vi "Set_Output.vi"(8 "error in (no error)":errorcluster caption="entrée d'erreur (pas d'erreur)", 10 "Output":string, 11 "Process (Default) en entrée":refnum<class "Process (Default).lvclass">) -> (0 "error out":errorcluster caption="sortie d'erreur", 3 "Process (Default) en sortie":refnum<class "Process (Default).lvclass">)   [LabVIEW 2020, in "Library Instrument & Equipement.lvlib" / "Process (Default).lvclass"]
uses:
  Process (Default).lvclass
  Process (Default).lvclass/Process (Default).ctl
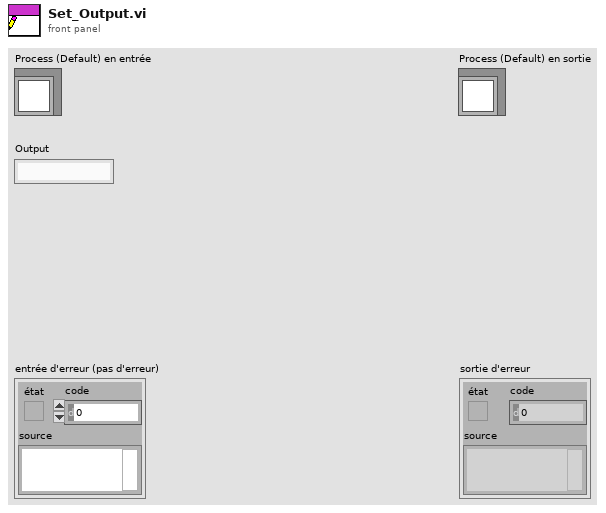
[diagram p1: front panel]
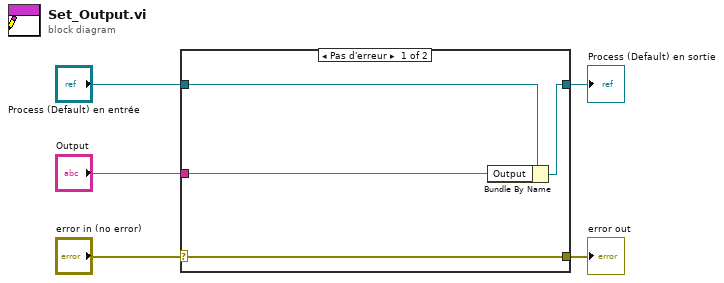
[diagram p0: block diagram]
diagram:
  n1 = case shown="Pas d'erreur" "error in (no error)" {
    selector: "error in (no error)" -> [w9 w10]
    tunnel: [w9 w10] -> w4
    tunnel: [w7 w11] -> w2
    tunnel: "Process (Default) en entrée" -> [w8 w11]
    tunnel: "Output" -> [w6 _]
    frame No Error {
      n2 = Bundle By Name(cluster=w8, "Output"=w6) -> (w7:refnum<class "Process (Default).lvclass">)
    }
    frame Error {
    }
  }
  "error out" <- w4
  "Process (Default) en sortie" <- w2
